vi "O to G peek.vi"(8 "height":dbl[](array[numeric]) format="%#_9g", 9 "south chip":dbl[](array[numeric]) format="%#_9g", 10 "north chip":dbl[](array[numeric]) format="%#_9g", 11 "Input file":path) -> (0 "OGP length":dbl format="%#_8g", 1 "output BR":dbl[](array[numeric]), 2 "output BL":dbl[](array[numeric]), 3 "output TL":dbl[](array[numeric]))   [LabVIEW 2016]
uses:
  <vilib>/Analysis/coordinate.llb/2D Cartesian Coordinate Rotation (Scalar).vi
  <vilib>/Utility/file.llb/Read Delimited Spreadsheet (DBL).vi
  <vilib>/Analysis/NI_AALPro.lvlib
panel:
  out "all rows":dbl[][](array[numeric])
  out "x+y":dbl[](array[numeric])
  out "Array":dbl[][](array[numeric]) format="%#_8g"
  out "south chip":dbl[](array[numeric]) format="%#_8g"
  out "north chip":dbl[](array[numeric]) format="%#_8g"
  out "south right":dbl[](array[numeric]) format="%#_8g"
  out "south left":dbl[](array[numeric])
  out "north left":dbl[](array[numeric])
  out "SC-NC":dbl[](array[numeric])
  out "rotation angle":dbl
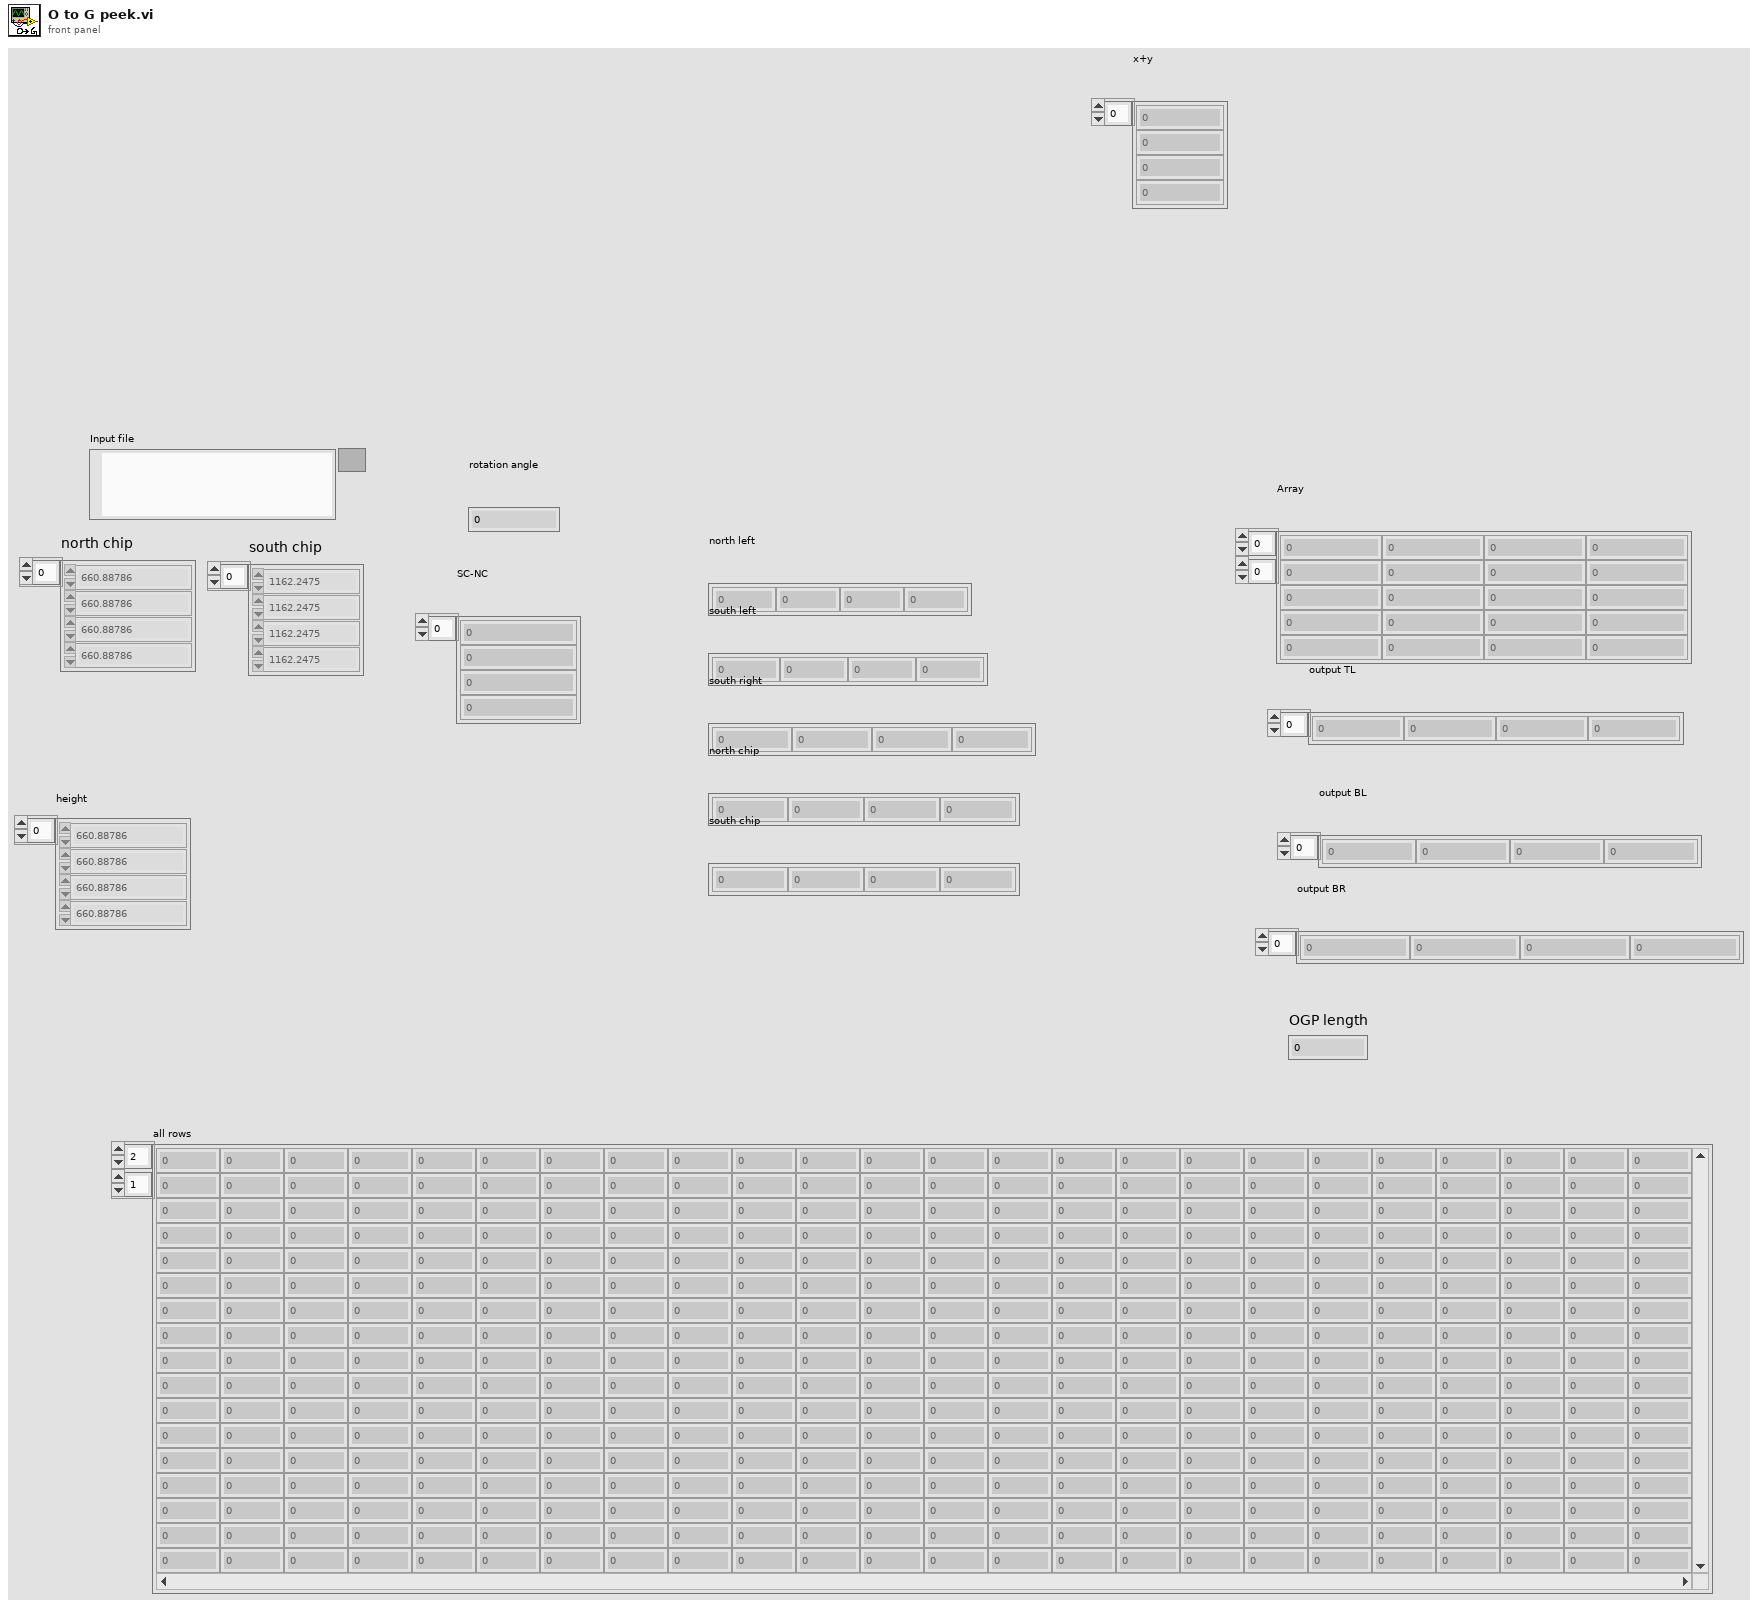
[diagram p1: front panel]
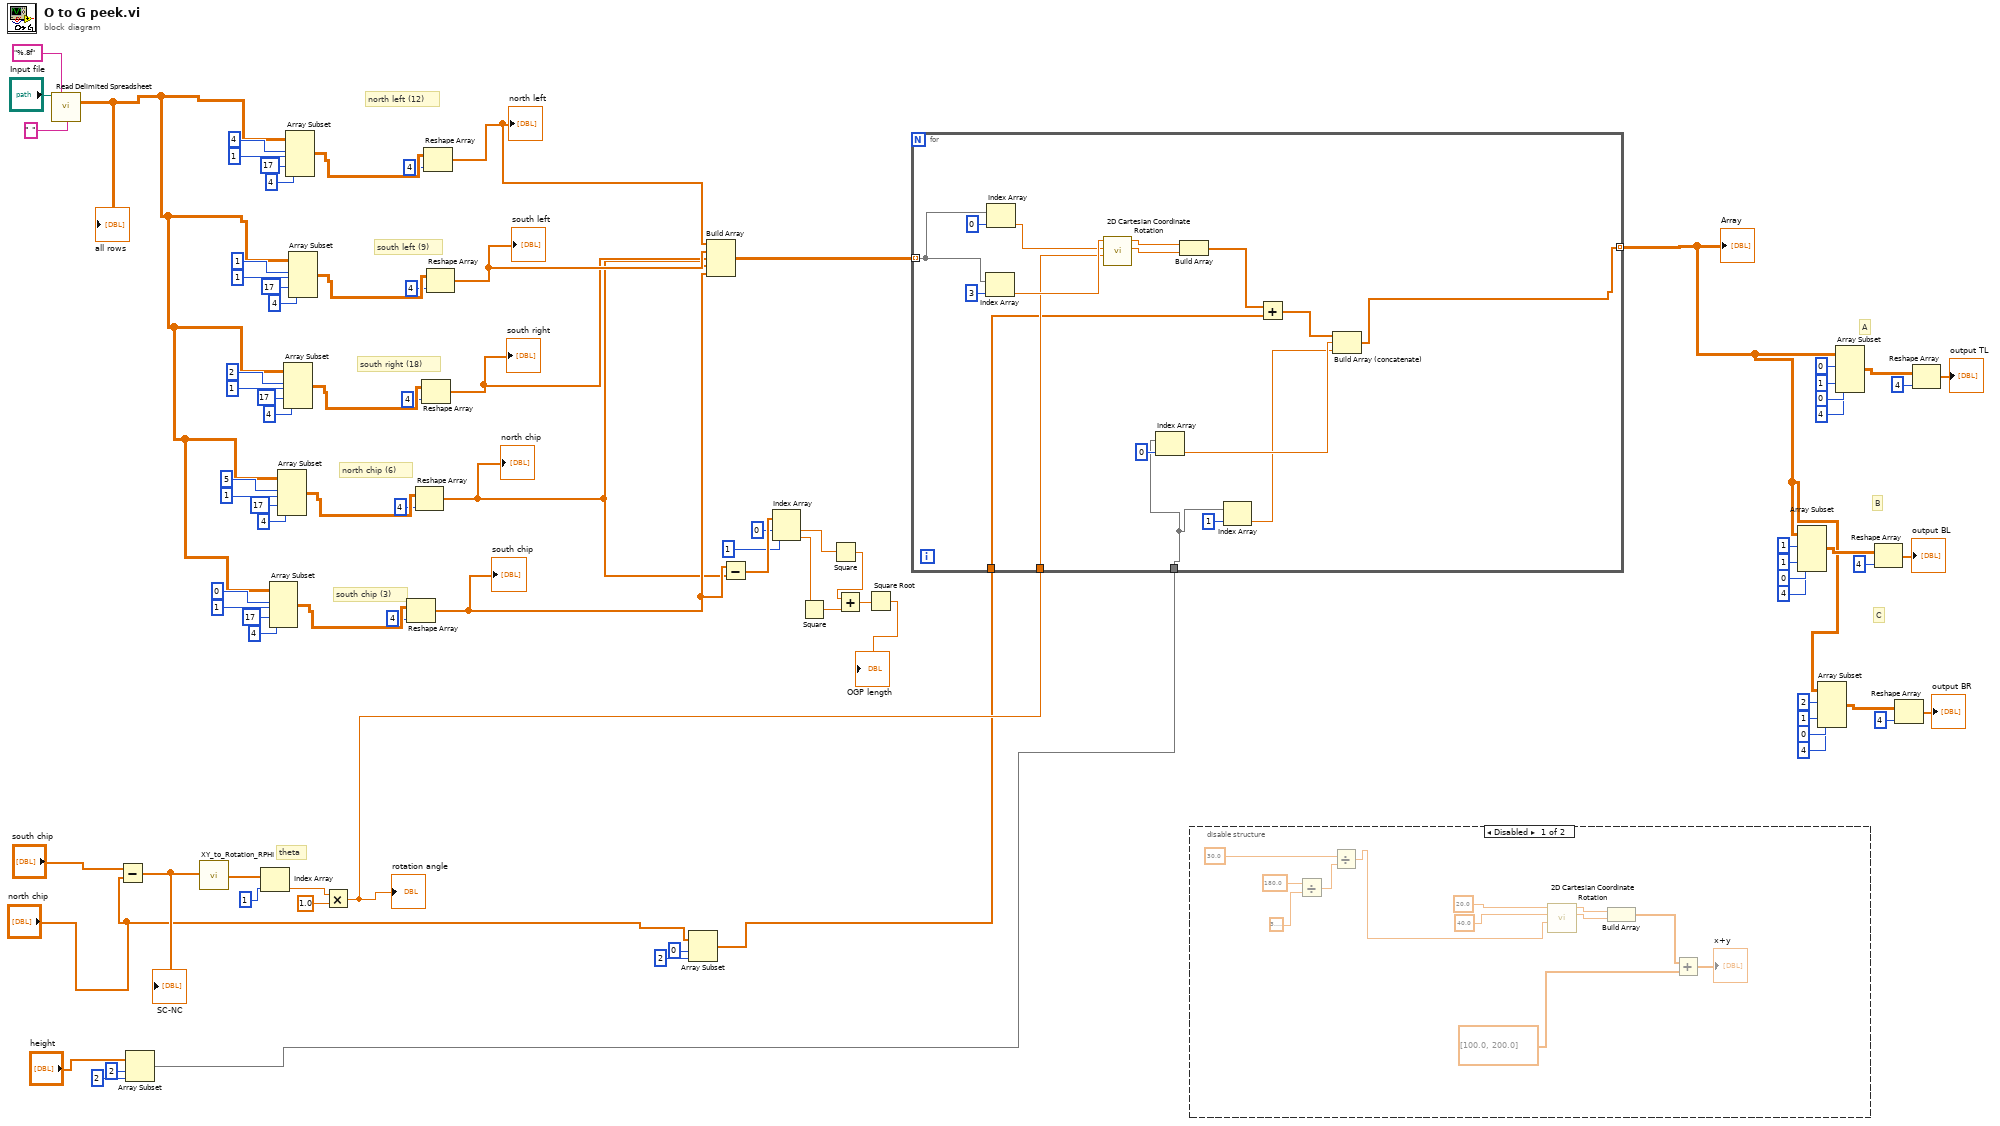
[diagram p0: block diagram]
diagram:
  # "C"
  # "B"
  # "A"
  # "south chip (3)"
  # "north chip (6)"
  # "south right (18)"
  # "south left (9)"
  # "north left (12)"
  # "theta"
  n1 = call-poly <vilib>:"Read Delimited Spreadsheet.vi"("file path (dialog if empty)"="Input file", "format (%.3f)"="%.8f", "delimiter (\\t)"=" " ("delimiter (\\t)")) -> ("all rows"=w49:dbl[][])  [unwired: 7 in, 5 out]
  "all rows" <- w49
  n2 = Subtract(x="south chip", y="north chip") -> (x-y=w80:dbl[])
  "SC-NC" <- w80
  n3 = Array Subset(array="height", index=2, length=2) -> (w38:dbl[])
  n4 = call "XY_to_Rotation_RPHI.vi"("X-Y"=w80) -> ("r-phi"=w83:dbl[])
  n5 = Index Array(array=w83, index=1) -> (element=w44:dbl)
  n6 = Array Subset(array=w49, index (row)=0 ("index"), length (row)=1 ("length"), index (col)=17 ("index"), length (col)=4 ("length")) -> (w51:dbl[][])
  n7 = Array Subset(array=w49, index (row)=5 ("index"), length (row)=1 ("length"), index (col)=17 ("index"), length (col)=4 ("length")) -> (w57:dbl[][])
  n8 = Array Subset(array=w49, index (row)=2 ("index"), length (row)=1 ("length"), index (col)=17 ("index"), length (col)=4 ("length")) -> (w63:dbl[][])
  n9 = Array Subset(array=w49, index (row)=4 ("index"), length (row)=1 ("length"), index (col)=17 ("index"), length (col)=4 ("length")) -> (w75:dbl[][])
  n10 = Array Subset(array=w49, index (row)=1 ("index"), length (row)=1 ("length"), index (col)=17 ("index"), length (col)=4 ("length")) -> (w69:dbl[][])
  n11 = Multiply(x=w44, y=1.0) -> (x*y=w43:dbl)
  "rotation angle" <- w43
  n12 = Reshape Array(w51, 4 ("dimension size")) -> (w3:dbl[])
  "south chip" <- w3
  n13 = Reshape Array(w57, 4 ("dimension size")) -> (w2:dbl[])
  "north chip" <- w2
  n14 = Reshape Array(w63, 4 ("dimension size")) -> (w46:dbl[])
  "south right" <- w46
  n15 = Reshape Array(w75, 4 ("dimension size")) -> (w48:dbl[])
  "north left" <- w48
  n16 = Reshape Array(w69, 4 ("dimension size")) -> (w47:dbl[])
  "south left" <- w47
  n17 = Array Subset(array="north chip", index=0, length=2) -> (w34:dbl[])
  n18 = Build Array(w48, w47, w46, w2, w3) -> (w45:dbl[][])
  n19 = Subtract(x=w3, y=w2) -> (x-y=w11:dbl[])
  n20 = Index Array(array=w11, index #1=0 ("index"), index #2=1 ("index")) -> (element #1=w8:dbl, element #2=w7:dbl)
  n21 = Square(x=w7) -> (x^2=w6:dbl)
  n22 = Square(x=w8) -> (x^2=w5:dbl)
  n23 = Add(x=w5, y=w6) -> (x+y=w4:dbl)
  n24 = Square Root(x=w4) -> (sqrt(x)=→"OGP length":dbl)
  n25 = for {
    tunnel: w45 -> [w101] mode=indexing
    tunnel: w43 -> [w98]
    tunnel: [w87] -> w12 mode=indexing
    tunnel: w34 -> [w95]
    tunnel: w38 -> [w90]
    n26 = Index Array(array=w101, index=3) -> (element=w100:dbl)
    n27 = Index Array(array=w101, index=0) -> (element=w99:dbl)
    n28 = call-poly <vilib>:"2D Cartesian Coordinate Rotation.vi"("theta"=w98, "y"=w99, "x"=w100) -> ("y out"=w96:dbl, "x out"=w97:dbl)  [unwired: 6 in, 1 out]
    n29 = Index Array(array=w90, index=0) -> (element=w89:dbl)
    n30 = Build Array(w97, w96) -> (w94:dbl[])
    n31 = Index Array(array=w90, index=1) -> (element=w88:dbl)
    n32 = Add(x=w94, y=w95) -> (x+y=w93:dbl[])
    n33 = Build Array (concatenate)(w93, w89, w88) -> (w87:dbl[])
  }
  "Array" <- w12
  n34 = disable-structure shown="Disabled" {
    frame Disabled {
      n35 = Divide(x=180.0, y=3.141592653589793) -> (x/y=w112:dbl)
      n36 = Divide(x=30.0, y=w112) -> (x/y=w109:dbl)
      n37 = call-poly <vilib>:"2D Cartesian Coordinate Rotation.vi"("theta"=w109, "y"=40.0, "x"=20.0) -> ("y out"=w107:dbl, "x out"=w108:dbl)  [unwired: 6 in, 1 out]
      n38 = Build Array(w108, w107) -> (w106:dbl[])
      n39 = Add(x=w106, y=dbl[] [100.0, 200.0]) -> (x+y=→"x+y":dbl[])
    }
    frame Enabled {
    }
  }
  n40 = Array Subset(array=w12, index (row)=1 ("index"), length (row)=1 ("length"), index (col)=0 ("index"), length (col)=4 ("length")) -> (w26:dbl[][])
  n41 = Array Subset(array=w12, index (row)=2 ("index"), length (row)=1 ("length"), index (col)=0 ("index"), length (col)=4 ("length")) -> (w19:dbl[][])
  n42 = Array Subset(array=w12, index (row)=0 ("index"), length (row)=1 ("length"), index (col)=0 ("index"), length (col)=4 ("length")) -> (w33:dbl[][])
  n43 = Reshape Array(w26, 4 ("dimension size")) -> (→"output BL":dbl[])
  n44 = Reshape Array(w19, 4 ("dimension size")) -> (→"output BR":dbl[])
  n45 = Reshape Array(w33, 4 ("dimension size")) -> (→"output TL":dbl[])
